vi "Handle Error.vi"(8 "error in (no error)":errorcluster, 11 "LoggingActor in":refnum<class "LoggingActor.lvclass">) -> (0 "error out":errorcluster, 2 "stop actor?":bool=TRUE, 3 "LoggingActor out":refnum<class "LoggingActor.lvclass">)   [LabVIEW 2022 SP3, in "LoggingActor.lvlib" / "LoggingActor.lvclass"]
doc: "(<B>Filename</B>: Actor Framework.lvlib:Actor.lvclass:Handle Error.vi)\n\nDefines how the actor handles an error that occurred while processing a message.\n\nBy default, this method does nothing except stop the actor. This method also treats error code 43 (coming from <B>error in</B>) as a sign that the actor shut down normally. In this situation, the Handle Error method does not return the error on <B>error out</B>, meaning the actor's caller will not receive it. All other error codes will be returned on <B>error out</B>.\n\nA descendant class may override this method to change this behavior."
uses:
  LoggingActor.lvclass
  LoggingActor.lvclass/LoggingActor.ctl
  Logger/Source/Logger/Logger.lvclass
  <vilib>/ActorFramework/Actor/Actor.lvclass
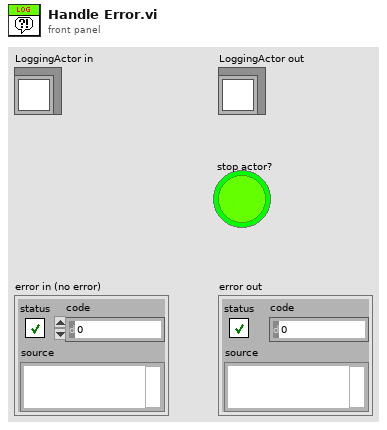
[diagram p1: front panel]
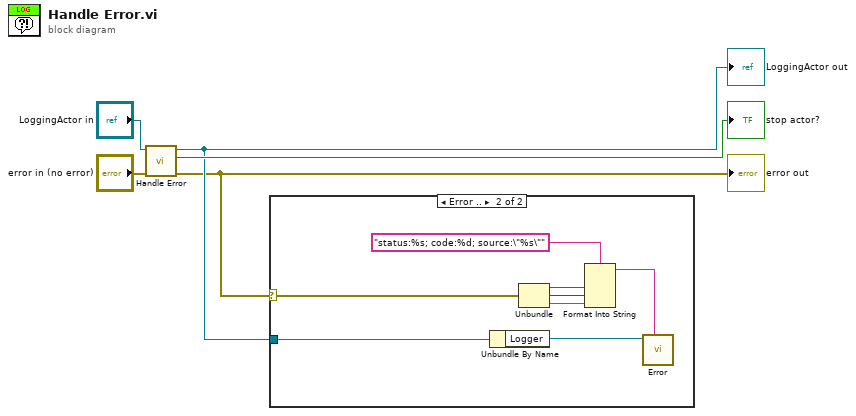
[diagram p0: block diagram]
diagram:
  n1 = call-parent "Handle Error.vi"("error in (no error)"="error in (no error)", "Actor in"="LoggingActor in") -> ("error out"=w1:errorcluster, "stop actor?"=→"stop actor?":bool, "Actor out"=w2:refnum<class "LoggingActor.lvclass">)  [unwired: 7 in]
  "LoggingActor out" <- w2
  "error out" <- w1
  n2 = case shown="Error .." w1 {
    selector: w1 -> [_ w6]
    tunnel: w2 -> [_ w13]
    frame No Error {
    }
    frame Error {
      n3 = Unbundle By Name(w13) -> ("Logger"=w12:refnum<class "Logger.lvclass">)
      n4 = Unbundle(w6) -> ("status"=w11:bool, "code"=w10:i32, "source"=w9:string)
      n5 = Format Into String(format string="status:%s; code:%d; source:\"%s\"", w11, w10, w9) -> (resulting string=w7:string)  [unwired: 2 in, 1 out]
      n6 = call-dynamic "Error.vi"("Message"=w7, "Logger in"=w12) -> ()  [unwired: 6 in, 2 out]
    }
  }
